vi "Prompt Convert 1.7 to 1.8.vi"(1 "Prompt 1.7 Test Parameters":T2) -> (0 "Prompt 1.8 Test Parameters":T1)   [LabVIEW 2011]
uses:
  TypeDefs/Prompt Test Parameters v1.7.ctl
  TypeDefs/Prompt Test Parameters v1.8.ctl
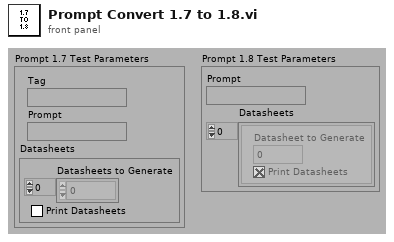
[diagram p1: front panel]
types:
  T1 = typedef "Prompt Test Parameters v1.8.ctl" = cluster{"Prompt":string, "Datasheets":cluster{"Datasheet to Generate":i32, "Print Datasheets":bool}[]}
  T2 = typedef "Prompt Test Parameters v1.7.ctl" = cluster{"Tag":string, "Prompt":string, "Datasheets":cluster{"Datasheets to Generate":i32[], "Print Datasheets":bool}}
  T3 = cluster{"Datasheet to Generate":i32, "Print Datasheets":bool}[]
  T4 = cluster{"Datasheet to Generate":i32, "Print Datasheets":bool}
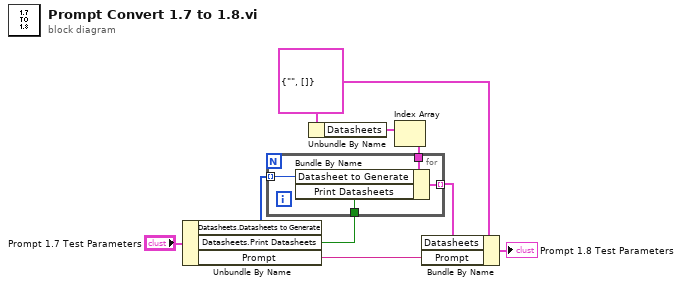
[diagram p0: block diagram]
diagram:
  w2 = T1 {"Prompt"="", "Datasheets"=[]} ("Prompt Test Parameters")
  n1 = Unbundle By Name("Prompt 1.7 Test Parameters") -> ("Datasheets.Datasheets to Generate"=w6:i32[], "Datasheets.Print Datasheets"=w5:bool, "Prompt"=w4:string)
  n2 = Unbundle By Name(w2) -> ("Datasheets"=w9:T3)
  n3 = Index Array(array=w9) -> (element=w8:T4)  [unwired: 1 in]
  n4 = for {
    tunnel: w8 -> [w13]
    tunnel: [w12] -> w3 mode=indexing
    tunnel: w6 -> [w11] mode=indexing
    tunnel: w5 -> [w10]
    n5 = Bundle By Name(cluster=w13, "Datasheet to Generate"=w11, "Print Datasheets"=w10) -> (w12:T4)
  }
  n6 = Bundle By Name(cluster=w2, "Datasheets"=w3, "Prompt"=w4) -> (→"Prompt 1.8 Test Parameters":T1)
